vi "Master FPGA Interface.vi"() -> ()   [LabVIEW 2011]
doc: "This VI shows an example of how to implement a closed loop position move using the NI 9505. The position loop is implemented using PID. The output of the loop is used as the command for the current loop, which then sets the PWM duty cycle for the motor. This example assumes that an encoder is connected for position and velocity feedback. This example does not implement advanced motion features such as trajectory generation and splining."
uses:
  <vilib>/LabVIEW Targets/FPGA/cRIO/cRIO-9505/controls.llb/_nicrio_cRIO-9505_DriveStatus.ctl
  <vilib>/Platform/TimedLoop/XDataNode/timing_clust.ctl
  <vilib>/Platform/TimedLoop/XDataNode/nitl_modes.ctl
  <vilib>/Platform/TimedLoop/XDataNode/wakeup.ctl
  <vilib>/LabVIEW Targets/FPGA/cRIO/cRIO-9505/controls.llb/_nicrio_cRIO-9505_DriveDirection.ctl
  Instance           1 55Saved   Position Control (closed loop) - NI 9505 (FPGA) .vi
  <vilib>/rvi/eio/common/nirviEmuTemplateMethod_errors.vi
  Instance           2 55Saved   Position Control (closed loop) - NI 9505 (FPGA) .vi
  <vilib>/rvi/eio/common/nirviEmuTemplatePropertyGet_noerrors.vi
  Instance           3 55Saved   Position Control (closed loop) - NI 9505 (FPGA) .vi
  <vilib>/Platform/TimedLoop/XDataNode/XDataNode.xnode
  <vilib>/eio/EIONode/EIONode.xnode
  <vilib>/eio/EIOMethodNode/EIOMethodNode.xnode
  <vilib>/eio/EIOPropertyNode/EIOPropertyNode.xnode
  <vilib>/Platform/TimedLoop/XDataNode/XDNodeRunTimeDep.lvlib
  <vilib>/rvi/eio/common/nirviEmuTemplatePropertyGet_errors.vi
  <vilib>/rvi/eio/common/nirviEmuTemplatePropertySet_errors.vi
  <vilib>/rvi/eio/common/nirviEmuTemplatePropertySet_noerrors.vi
panel:
  in  "Current Setpoint":i16
  out "Vsup Present":bool
  out "Drive Fault":bool
  out "Drive Status":T1=enum."Disabled"
  out "Temp Fault":bool
  in  "Enable\nDrive":bool
  in  "Disable\nDrive":bool
  in  "Reset Position":bool
  in  "Reset Position Value":i32
  out "Encoder Position":i32
  out "ticks/count":u32
  out "Index (Z) Position":i32
  out "counts (no reset)":i32
  in  "Current PI Gains":T2={"Proportional Gain"=20, "Integral Gain"=10, "Derivative Gain"=0}
  in  "Current Limit":i16 caption="Setpoint"
  in  "Current Loop\nRate (usec)":u32=50
  in  "Trig AI":bool
  in  "Current Feedback":i16
  out "Current Loop Output":i16
  # "VI Execution\nThis VI should be run with \"Position Control (closed loop) - NI 9505 (RT).vi\"."
  # "These parameters control the response of the position loop. Position Setpoint is the desired position to go to. Position Error Limit is the maximum allowed error the setpoint and actual position returned by the encoder loop."
  # "These parameters control the response\nof the current loop. The current limit is the \nmaximum current allowed."
  # "Current Loop Parameters"
  # "Use the Reset Position control to reset the quadrature count to the value in Reset Position Value."
  # "These status controls/indicators are used to enable/disable the drive and read fault information."
  # "Drive Status"
  # "Encoder Parameters"
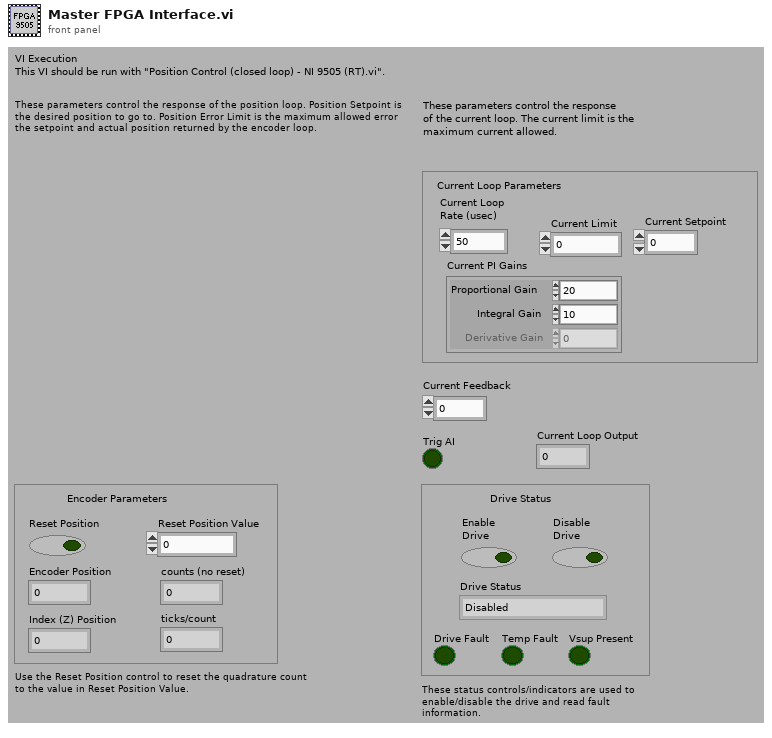
[diagram p1: front panel]
types:
  T1 = typedef "_nicrio_cRIO-9505_DriveStatus.ctl" = enum8{"Enabled", "Disabled", "Disabled by Drive Fault", "Disabled by Temp. Fault", "Disabled by E-Stop", "Unknown"}
  T2 = cluster{"Proportional Gain":i16, "Integral Gain":i16, "Derivative Gain":i16}
  T3 = typedef "XDNodeRunTimeDep.lvlib/timing_clust.ctl" = cluster{"Expected End [f-1]":u64, "Actual End [f-1]":u64, "Finished Late? [f-1]":bool, "Expected End [i-1]":u64, "Actual End [i-1]":u64, "Finished Late? [i-1]":bool, "Expected Start [i]":u64, "Actual Start [i]":u64, "Expected Start [f]":u64, "Actual Start [f]":u64, "Source Name":string, "Structure Name":string, "Period":i64, "Deadline":i64, "Offset":i64, "Start":i64, "Priority":i32, "Timeout":i32, "Mode":T4, "Wakeup Reason":T5, "Error":errorcluster, "Source Type":string, "Secondary Source Type":string, "Global End Time":u64, "Global Start Time":u64, "Frame Duration":u64, "Iteration Duration":u64, "Assigned CPU":i32, "I/O Scan Engine Mode":u32}
  T4 = typedef "XDNodeRunTimeDep.lvlib/nitl_modes.ctl" = enum32{"No Change", "Process missed periods, maintain original phase", "Discard missed periods, maintain original phase", "Process missed periods, ignore original phase", "Discard missed periods, ignore original phase"}
  T5 = typedef "XDNodeRunTimeDep.lvlib/wakeup.ctl" = enum32{"Normal", "Aborted", "Asynchronous wakeup", "Timing source error", "Timed loop error", "Timeout"}
  T6 = typedef "_nicrio_cRIO-9505_DriveDirection.ctl" = enum8{"Clockwise", "Counterclockwise"}
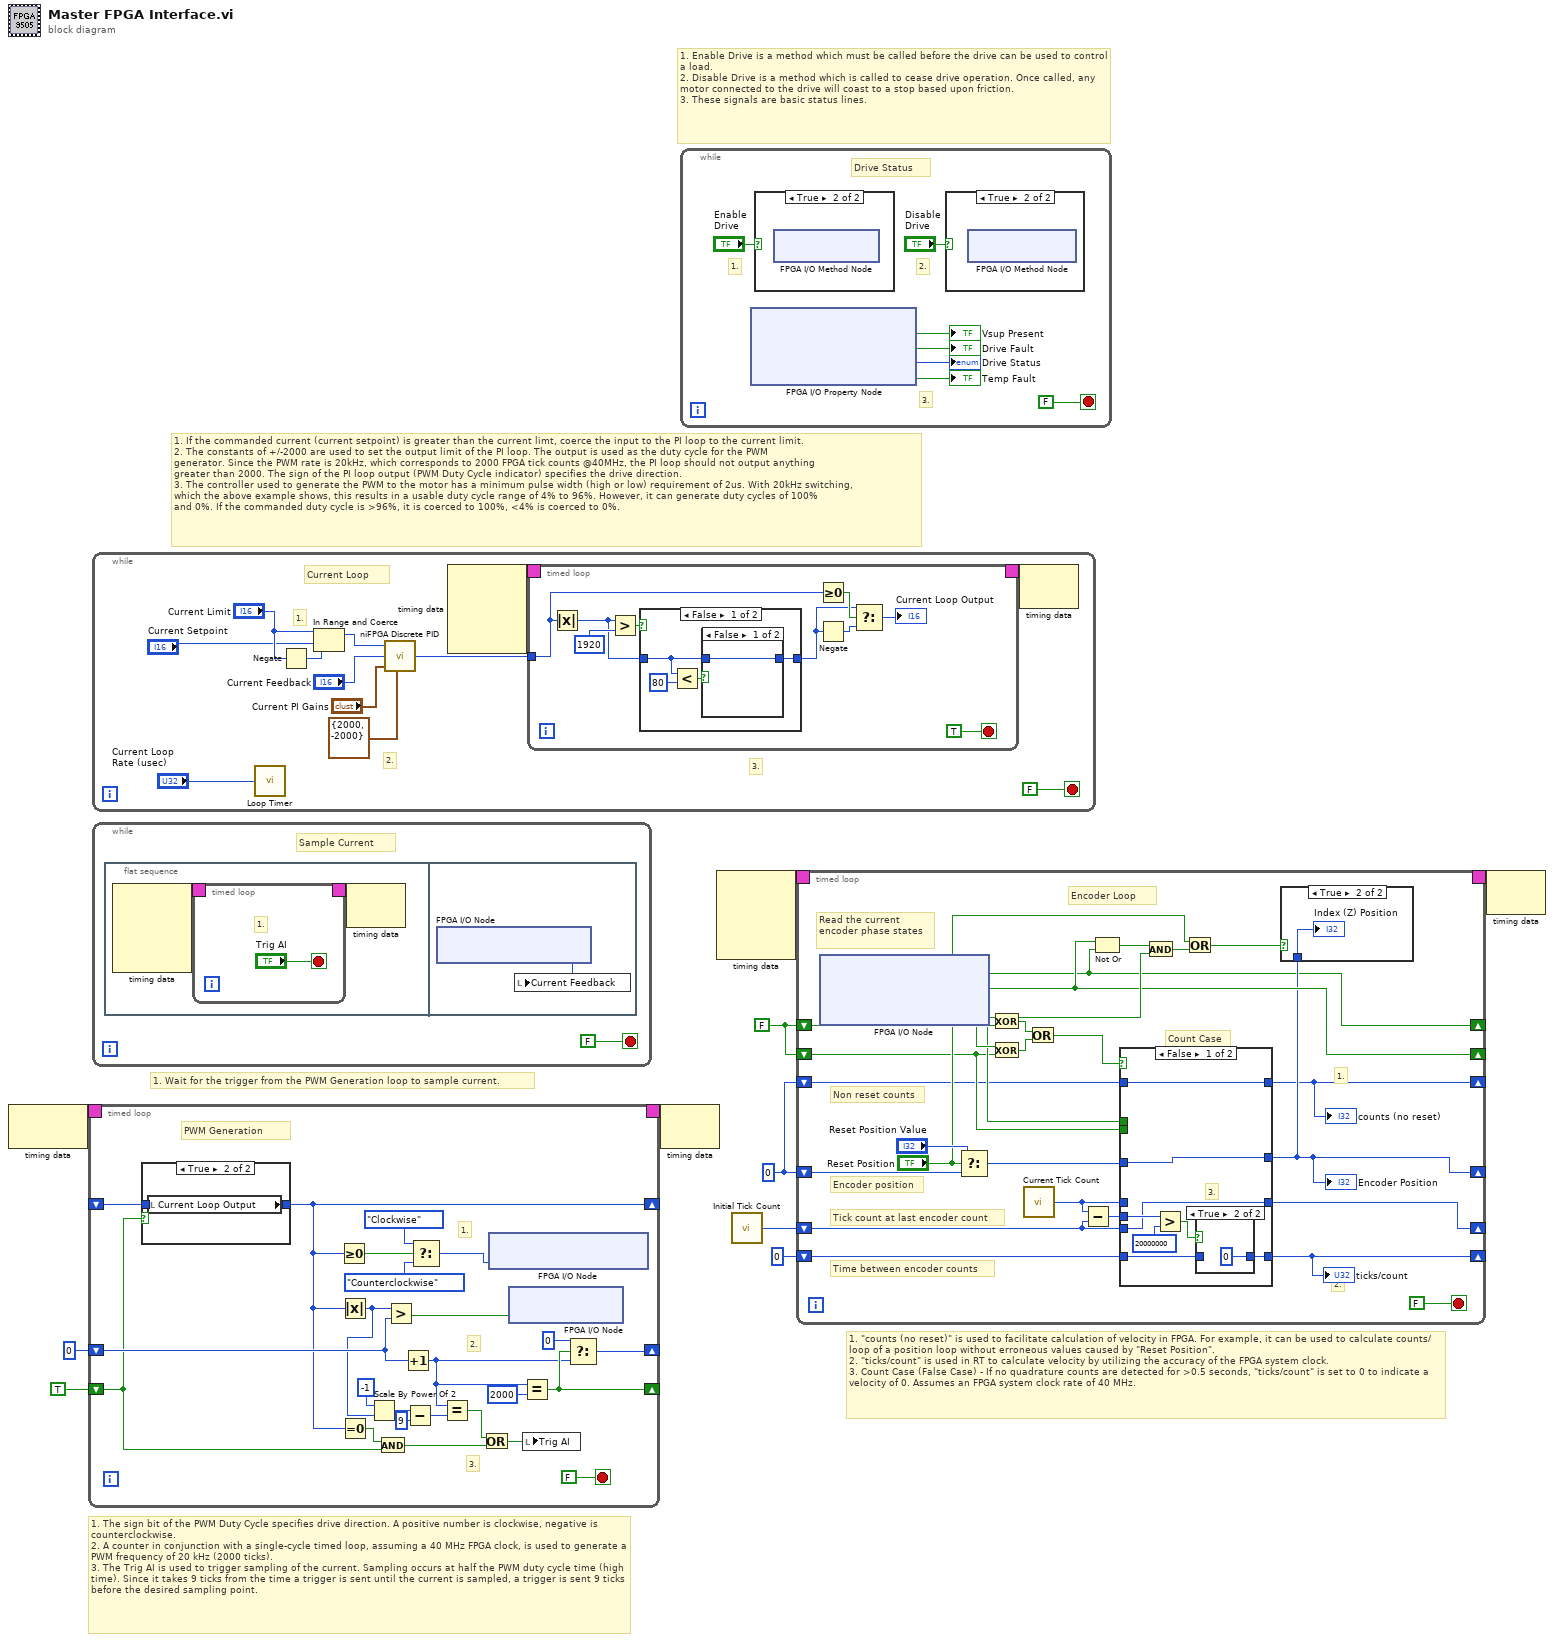
[diagram p0: block diagram]
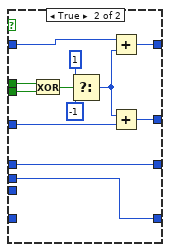
[diagram p4: hidden frame]
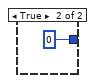
[diagram p6: hidden frame]
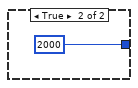
[diagram p7: hidden frame]
diagram:
  w1 = 0 ("Reset Position Value")
  w4 = FALSE ("Encoder Phase A")
  # "1. \"counts (no reset)\" is used to facilitate calculation of velocity in FPGA. For example, it can be used to calculate counts/loop of a position loop without erroneous values caused by \"Reset Position\". \n2. \"ticks/count\" is used in RT to calculate velocity by utilizing the accuracy of the FPGA system clock.\n3. Count Case (False Case) - If no quadrature counts are detected for >0.5 seconds, \"ticks/count\" is set to 0 to indicate a velocity of 0. Assumes an FPGA system clock rate of 40 MHz."
  # "1. Enable Drive is a method which must be called before the drive can be used to control a load.\n2. Disable Drive is a method which is called to cease drive operation. Once called, any motor connected to the drive will coast to a stop based upon friction.\n3. These signals are basic status lines."
  # "1. The sign bit of the PWM Duty Cycle specifies drive direction. A positive number is clockwise, negative is counterclockwise. \n2. A counter in conjunction with a single-cycle timed loop, assuming a 40 MHz FPGA clock, is used to generate a PWM frequency of 20 kHz (2000 ticks).\n3. The Trig AI is used to trigger sampling of the current. Sampling occurs at half the PWM duty cycle time (high time). Since it takes 9 ticks from the time a trigger is sent until the current is sampled, a trigger is sent 9 ticks before the desired sampling point."
  # "1. Wait for the trigger from the PWM Generation loop to sample current."
  # "1. If the commanded current (current setpoint) is greater than the current limt, coerce the input to the PI loop to the current limit.\n2. The constants of +/-2000 are used to set the output limit of the PI loop. The output is used as the duty cycle for the PWM\ngenerator. Since the PWM rate is 20kHz, which corresponds to 2000 FPGA tick counts @40MHz, the PI loop should not output anything\ngreater than 2000. The sign of the PI loop output (PWM Duty Cycle indicator) specifies the drive direction.\n3. The controller used to generate the PWM to the motor has a minimum pulse width (high or low) requirement of 2us. With 20kHz switching,\nwhich the above example shows, this results in a usable duty cycle range of 4% to 96%. However, it can generate duty cycles of 100%\nand 0%. If the commanded duty cycle is >96%, it is coerced to 100%, <4% is coerced to 0%."
  n1 = node-c288() -> (w10:T3)  [unwired: 1 out]
  n2 = timed-loop {
    timing: w10 -> [_]
    timing-out: [_] -> w9
    shift-right: [w31] -> _
    shift-left: i16 0 -> [w34]
    shift-right: [w30] -> _
    shift-left: TRUE -> [w27]
    shift-right: [w15] -> _
    shift-left: _ -> [w29]
    stop <- FALSE stop-if-true
    # "3."
    # "2."
    # "1."
    # "PWM Generation"
    n3 = case shown="True" w27 {
      tunnel: [w35 w36] -> w15
      tunnel: w29 -> [w35 _]
      frame False {
      }
      frame True {
        n4 = local read "Current Loop Output"() -> (w36:i16)
      }
    }
    n5 = Greater Or Equal To 0?(x=w15) -> (x >= 0?=w23:bool)
    n6 = Absolute Value(x=w15) -> (abs(x)=w13:i16)
    n7 = Equal To 0?(x=w15) -> (x = 0?=w28:bool)
    n8 = Scale By Power Of 2(n=i8 -1, x=w13) -> (x*2^n=w17:i16)
    n9 = And(x=w28, y=w27) -> (x .and. y?=w24:bool)
    n10 = Greater?(x=w13, y=w34) -> (0:w12:bool)
    n11 = Increment(x=w34) -> (x+1=w26:i16)
    n12 = Subtract(x=w17, y=i8 9) -> (x-y=w16:i16)
    n13 = Select(t=_nicrio_cRIO-9505_DriveDirection."Clockwise" ("Drive Direction"), s=w23, f=_nicrio_cRIO-9505_DriveDirection."Counterclockwise" ("Drive Direction")) -> (s? t:f=w11:T6)
    n14 = Equal?(x=w26, y=w16) -> (x = y?=w25:bool)
    n15 = Or(x=w25, y=w24) -> (x .or. y?=w19:bool)
    n16 = xnode "FPGA I/O Node"("Motor/Drive Direction"=w11) -> ()  [unwired: 1 in, 1 out]
    n17 = xnode "FPGA I/O Node"("Motor/Motor"=w12) -> ()  [unwired: 1 in, 1 out]
    n18 = Equal?(x=w26, y=i16 2000) -> (x = y?=w30:bool)
    n19 = local write "Trig AI"(w19) -> ()
    n20 = Select(t=i16 0, s=w30, f=w26) -> (s? t:f=w31:i16)
  }
  n21 = while {
    stop <- FALSE stop-if-true
    # "3."
    # "2."
    # "1."
    # "Current Loop"
    n22 = call "Loop Timer"("Count(uSec)"="Current Loop\nRate (usec)") -> ()  [unwired: 1 out]
    n23 = Negate(x="Current Limit") -> (-x=w43:i16)
    n24 = In Range and Coerce(upper limit="Current Limit", x="Current Setpoint", lower limit=w43) -> (coerced(x)=w41:i16)  [unwired: 1 out]
    n25 = call <vilib>:"niFPGA Discrete PID.vi"("setpoint"=w41, "process variable"="Current Feedback", "PID gains (x 2^8)"="Current PI Gains", "output range"=cluster{"output high":i16, "output low":i16} {"output high"=2000, "output low"=-2000}) -> ("output"=w46:i16)  [unwired: 1 in, 4 out]
    n26 = node-c288() -> (w45:T3)  [unwired: 4 out]
    n27 = timed-loop {
      timing: w45 -> [_]
      timing-out: [_] -> w44
      tunnel: w46 -> [w53]
      stop <- TRUE stop-if-true
      n28 = Absolute Value(x=w53) -> (abs(x)=w54:i16)
      n29 = Greater?(x=w54, y=i16 1920 ("upper limit")) -> (0:w56:bool)
      n30 = case shown="False" w56 {
        tunnel: [w62 i16 2000 ("upper limit")] -> w55
        tunnel: w54 -> [w60 _]
        frame False {
          n31 = Less?(x=w60, y=i16 80 ("lower limit")) -> (x < y?=w61:bool)
          n32 = case shown="False" w61 {
            tunnel: [w64 i16 0 ("upper limit")] -> w62
            tunnel: w60 -> [w64 _]
            frame False {
            }
            frame True {
            }
          }
        }
        frame True {
        }
      }
      n33 = Greater Or Equal To 0?(x=w53) -> (x >= 0?=w59:bool)
      n34 = Negate(x=w55) -> (-x=w58:i16)
      n35 = Select(t=w55, s=w59, f=w58) -> (s? t:f=→"Current Loop Output":i16)
    }
    n36 = node-c288(w44) -> ()  [unwired: 1 out]
  }
  n37 = while {
    stop <- FALSE stop-if-true
    # "Sample Current"
    n38 = flat-sequence {
      frame #0 {
        n39 = node-c288() -> (w73:T3)  [unwired: 4 out]
        n40 = timed-loop {
          timing: w73 -> [_]
          timing-out: [_] -> w72
          stop <- "Trig AI" stop-if-true
          # "1."
        }
        n41 = node-c288(w72) -> ()  [unwired: 1 out]
      }
      frame #1 {
        n42 = xnode "FPGA I/O Node"() -> ("Motor/Current Sense"=w79:i16)  [unwired: 1 in, 1 out]
        n43 = local write "Current Feedback"(w79) -> ()
      }
    }
  }
  n44 = node-c288(w9) -> ()  [unwired: 1 out]
  n45 = while {
    stop <- FALSE stop-if-true
    # "Drive Status"
    # "3."
    # "2."
    # "1."
    n46 = xnode "FPGA I/O Property Node"() -> ("Vsup Present"=→"Vsup Present":bool, "Drive Fault"=→"Drive Fault":bool, "Drive Status"=→"Drive Status":T1, "Over Temperature Fault"=→"Temp Fault":bool)  [unwired: 1 in, 1 out]
    n47 = case shown="True" "Enable\nDrive" {
      frame False {
      }
      frame True {
        n48 = xnode "FPGA I/O Method Node"() -> ()  [unwired: 1 in, 1 out]
      }
    }
    n49 = case shown="True" "Disable\nDrive" {
      frame False {
      }
      frame True {
        n50 = xnode "FPGA I/O Method Node"() -> ()  [unwired: 1 in, 1 out]
      }
    }
  }
  n51 = node-c288() -> (w6:T3)  [unwired: 4 out]
  n52 = call "Initial Tick Count"() -> ("Tick Count(Ticks)"=w3:u32)
  n53 = timed-loop {
    shift-right: [w93] -> _
    shift-left: w4 -> [w111]
    shift-right: [w99] -> _
    shift-left: w4 -> [w92]
    shift-right: [w95] -> _
    shift-left: w1 -> [w108]
    shift-right: [w104] -> _
    shift-left: w3 -> [w88]
    shift-right: [w103] -> _
    shift-left: u32 0 -> [w102]
    timing: w6 -> [_]
    timing-out: [_] -> w5
    shift-right: [w90] -> _
    shift-left: w1 -> [w91]
    stop <- FALSE stop-if-true
    # "Count Case"
    # "Encoder Loop"
    # "2."
    # "1."
    # "Read the current\nencoder phase states"
    # "Non reset counts"
    # "Encoder position"
    # "Time between encoder counts"
    # "Tick count at last encoder count"
    n54 = xnode "FPGA I/O Node"() -> ("Motor/Encoder Phase A"=w93:bool, "Motor/Encoder Phase B"=w99:bool, "Motor/Encoder Index"=w100:bool)  [unwired: 3 in, 3 out]
    n55 = Select(t="Reset Position Value", s="Reset Position", f=w108) -> (s? t:f=w106:i32)
    n56 = Exclusive Or(1:w111, 2:w93) -> (0:w110:bool)
    n57 = Exclusive Or(1:w92, 2:w99) -> (0:w109:bool)
    n58 = call "Current Tick Count"() -> ("Tick Count(Ticks)"=w89:u32)
    n59 = Or(x=w110, y=w109) -> (x .or. y?=w107:bool)
    n60 = Subtract(x=w89, y=w88) -> (x-y=w87:u32)
    n61 = Not Or(1:w93, 2:w99) -> (0:w97:bool)
    n62 = case shown="False" w107 {
      tunnel: [w120 w128] -> w95
      tunnel: w106 -> [w120 w134]
      tunnel: w89 -> [_ w124]
      tunnel: [w115 w124] -> w104
      tunnel: w88 -> [w115 _]
      tunnel: [w113 w123] -> w103
      tunnel: w102 -> [w114 _]
      tunnel: w93 -> [_ w130]
      tunnel: w92 -> [_ w129]
      tunnel: [w119 w126] -> w90
      tunnel: w91 -> [w119 w125]
      tunnel: w87 -> [w116 w123]
      frame False {
        # "3."
        n63 = Greater?(x=w116, y=20000000 ("x")) -> (0:w117:bool)
        n64 = case shown="True" w117 {
          tunnel: [w121 u32 0] -> w113
          tunnel: w114 -> [w121 _]
          frame False {
          }
          frame True {
          }
        }
      }
      frame True {
        n65 = Exclusive Or(1:w129, 2:w130) -> (0:w131:bool)
        n66 = Select(t=1 ("16 bit"), s=w131, f=-1 ("16 bit")) -> (s? t:f=w127:i32)
        n67 = Add(x=w125, y=w127) -> (x+y=w126:i32)
        n68 = Add(x=w127, y=w134) -> (x+y=w128:i32)
      }
    }
    "Encoder Position" <- w95
    "ticks/count" <- w103
    "counts (no reset)" <- w90
    n69 = And(x=w97, y=w100) -> (x .and. y?=w98:bool)
    n70 = Or(x="Reset Position", y=w98) -> (x .or. y?=w96:bool)
    n71 = case shown="True" w96 {
      tunnel: w95 -> [_ w112]
      frame False {
      }
      frame True {
        "Index (Z) Position" <- w112
      }
    }
  }
  n72 = node-c288(w5) -> ()  [unwired: 1 out]
